vi "Test_Register Service.vi"() -> ()   [LabVIEW 2020]
uses:
  Discovery_client/RPC Messages/ni_measurements_discovery_v1_RegisterServiceResponse.ctl
  Discovery_client/RPC Messages/ni_measurements_discovery_v1_RegisterServiceRequest.ctl
  Discovery_client/RPC Messages/ni_measurements_discovery_v1_ServiceDescriptor.ctl
  Discovery_client/RPC Messages/ni_measurements_discovery_v1_ServiceLocation.ctl
  Discovery_client/Discovery_client.lvlib
panel:
  out "Response Data":T1
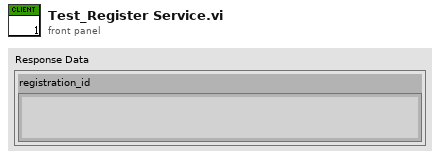
[diagram p1: front panel]
types:
  T1 = typedef "Discovery_client.lvlib/ni_measurements_discovery_v1_RegisterServiceResponse.ctl" = cluster{"registration_id":string}
  T2 = typedef "Discovery_client.lvlib/ni_measurements_discovery_v1_RegisterServiceRequest.ctl" = cluster{"service_description":T3, "provided_services":string[], "location":T4}
  T3 = typedef "Discovery_client.lvlib/ni_measurements_discovery_v1_ServiceDescriptor.ctl" = cluster{"service_id":string, "name":string, "description_url":string, "service_class":string}
  T4 = typedef "Discovery_client.lvlib/ni_measurements_discovery_v1_ServiceLocation.ctl" = cluster{"location":string, "optimal_route":string, "insecure_port":string, "ssl_authenticated_port":string}
  T5 = typedef "gprc-lvsupport-release.lvlib/grpcId.ctl" = u64
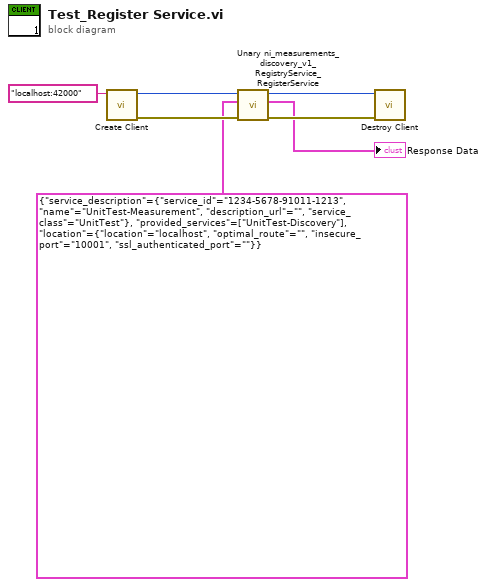
[diagram p0: block diagram]
diagram:
  n1 = call "Create Client.vi"("address"="localhost:42000") -> ("error out"=w5:errorcluster, "gRPC ID Out"=w6:T5)  [unwired: 9 in]
  n2 = call "Unary ni_measurements_discovery_v1_RegistryService_RegisterService.vi"("error in"=w5, "Request Data"=T2 {"service_description"={"service_id"="1234-5678-91011-1213", "name"="UnitTest-Measurement", "description_url"="", "service_class"="UnitTest"}, "provided_services"=["UnitTest-Discovery"], "location"={"location"="localhost", "optimal_route"="", "insecure_port"="10001", "ssl_authenticated_port"=""}}, "gRPC ID"=w6) -> ("error out"=w4:errorcluster, "Response Data"=→"Response Data":T1, "gRPC ID out"=w3:T5)  [unwired: 6 in]
  n3 = call "Destroy Client.vi"("error in"=w4, "gRPC ID"=w3) -> ()  [unwired: 9 in, 1 out]
